vi "Generate RAW Frame.vi"(8 "error in (no error)":errorcluster, 10 "Data to Send":T1 {"Identifier" format="%08x"}, 11 "Connection Info":T2) -> (0 "error out":errorcluster, 3 "Connection Info Out":T2)   [LabVIEW 2015, in "J1939 Addon Shared.lvlib"]
uses:
  J1939 Addon Shared.lvlib
  STM/TCP/stm_TCP Connection Info.ctl
  STM/_SubVIs/stm_MetaDataElement.ctl
  J1939 Utilities/Types/CAN Outgoing Message Cluster.ctl
  J1939 Utilities/J1939 Utilities.lvlib
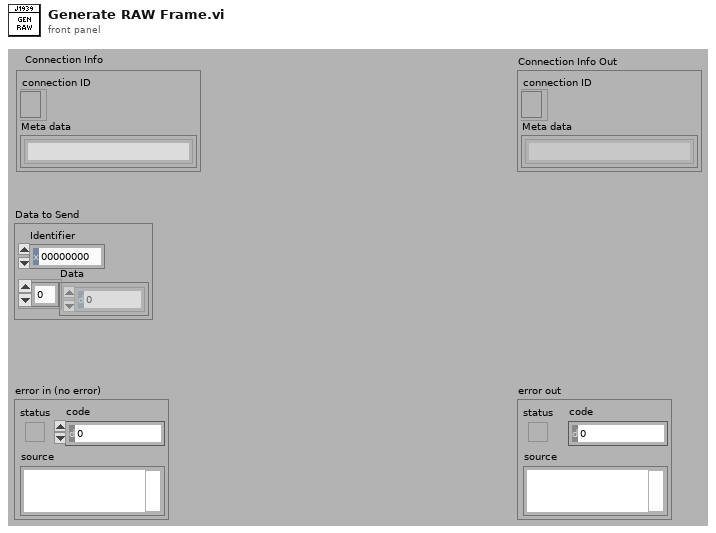
[diagram p1: front panel]
types:
  T1 = typedef "J1939 Addon Shared.lvlib/J1939 Utilities.lvlib/CAN Outgoing Message Cluster.ctl" = cluster{"Identifier":u32, "Data":u8[]}
  T2 = typedef "J1939 Addon Shared.lvlib/stm_TCP Connection Info.ctl" = cluster{"connection ID":refnum<k5>, "Meta data":T3[]}
  T3 = typedef "J1939 Addon Shared.lvlib/stm_MetaDataElement.ctl" = string
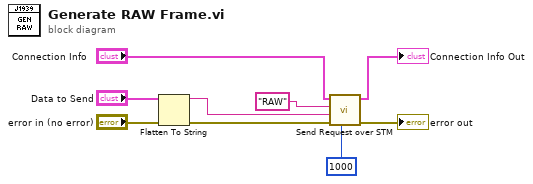
[diagram p0: block diagram]
diagram:
  n1 = Flatten To String(anything="Data to Send", error in (no error)="error in (no error)") -> (data string=w5:string, error out=w1:errorcluster)  [unwired: 2 in, 1 out]
  n2 = call "Send Request over STM.vi"("Timeout (ms)"=1000 ("Timeout ms (5000)"), "error in (no error)"=w1, "Data"=w5, "Name"="RAW" ("Command"), "Connection Info"="Connection Info") -> ("error out"=→"error out":errorcluster, "Connection Info Out"=→"Connection Info Out":T2)  [unwired: 3 in, 2 out]
